vi "Video feed info class VI - states.vi"(0 "Video feed info in":refnum<class "Video feed info.lvclass">, 1 "States":T1, 2 "start path":path, 4 "Start/Stop":bool, 5 "error in (no error)":errorcluster, 6 "Slide Refnum":refnum<vi>) -> (8 "Image":T3(plugin-control), 9 "Start/Stop output":bool, 10 "file path":path, 11 "State output":T2(ring), 12 "Image Type":T4 items=["Grayscale (U8)", "Grayscale (I16)", "Grayscale (SGL)", "Complex (CSG)", "RGB (U32)", "HSL (U32)", "RGB (U64)", "Grayscale (U16)"], 13 "Current Frame":u32, 14 "Video feed info out":refnum<class "Video feed info.lvclass">, 15 "FPS":u32, 16 "width":u32, 17 "height":u32, 18 "Number of Frames":u32, 19 "error out":errorcluster)   [LabVIEW 2010, in "Video feed info.lvclass"]
uses:
  Video feed info.lvclass
  Controls/video control.ctl
  <vilib>/Vision/Image Controls.llb/IMAQ Image.ctl
  Video feed info.lvclass/Video feed info.ctl
  <vilib>/vision/Avi1.llb/AviRefnum.ctl
  <vilib>/vision/NI_Vision_Development_Module.lvlib
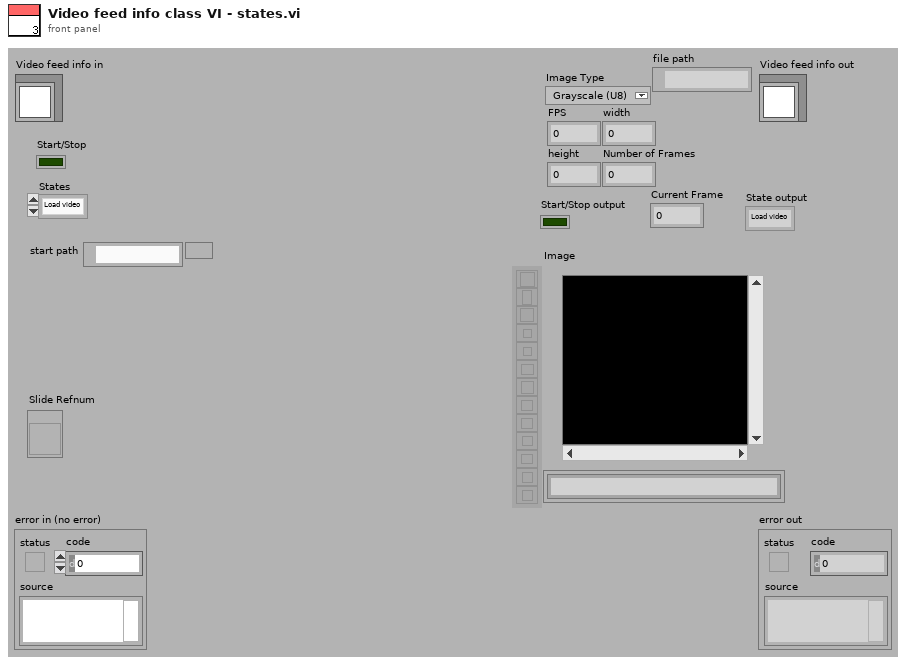
[diagram p1: front panel]
types:
  T1 = typedef "video control.ctl" = enum16{"Load video", "Idle", "Play", "Rewind", "Forward", "Dispose"}
  T2 = enum16{"Load video", "Idle", "Play", "Rewind", "Forward", "Dispose"}
  T3 = typedef "IMAQ Image.ctl" = refnum<image>
  T4 = typedef "Image Type" = u32
  T5 = cluster{"Number of Frames":u32, "Number of Frames":u32, "Number of Frames":u32}
  T6 = typedef "AviRefnum.ctl" = refnum<k1>
  T7 = cluster{"width":u32, "height":u32, "framesPerSecond":u32, "compressionFilter":string, "hasData":bool}
  T8 = cluster{"Higher Cursor value":u32, "Lower Cursor value":u32, "Current Frame":u32}
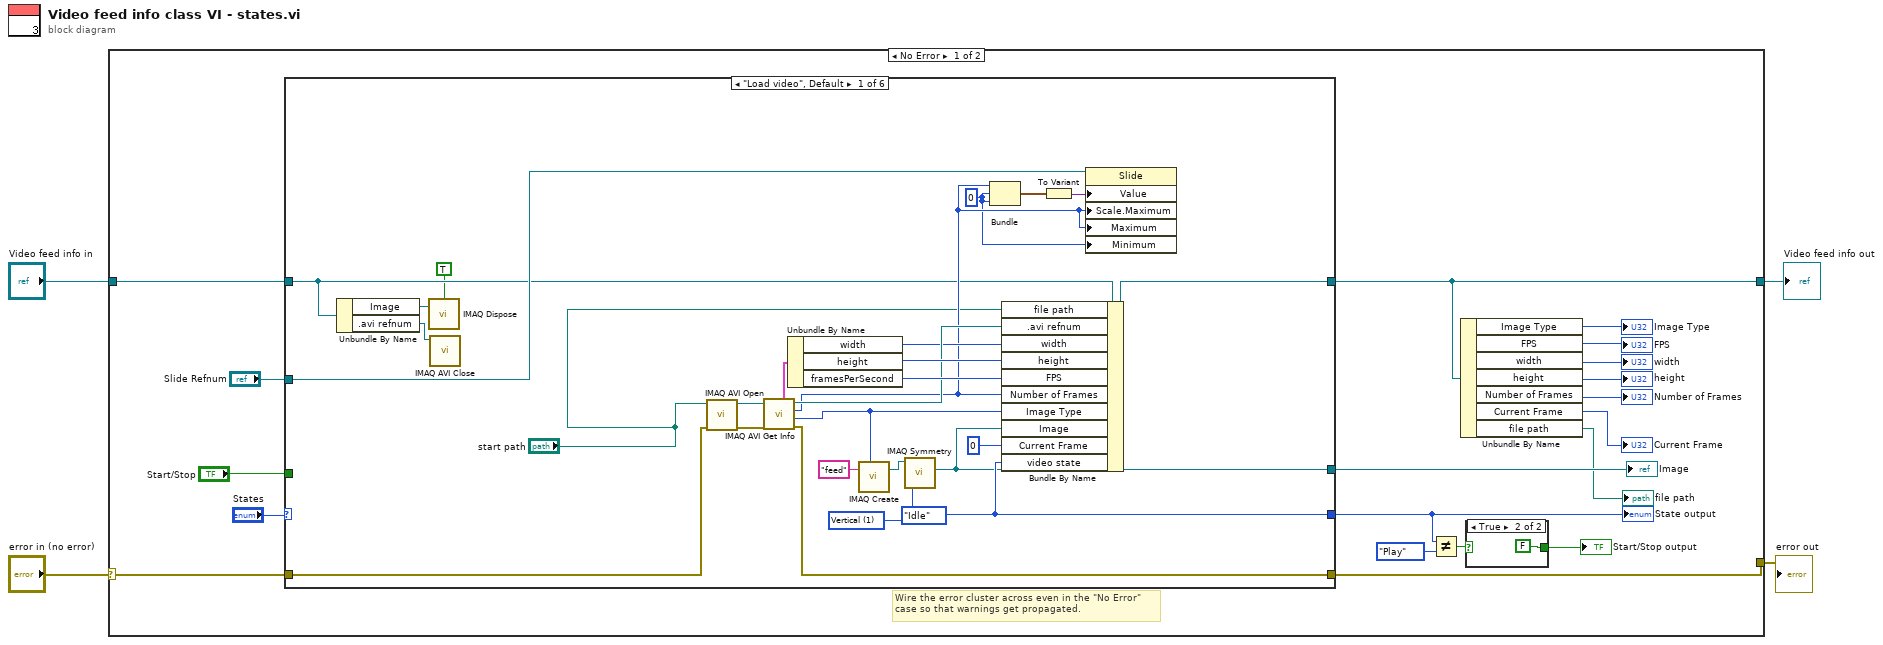
[diagram p0: block diagram]
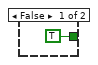
[diagram p2: hidden frame]
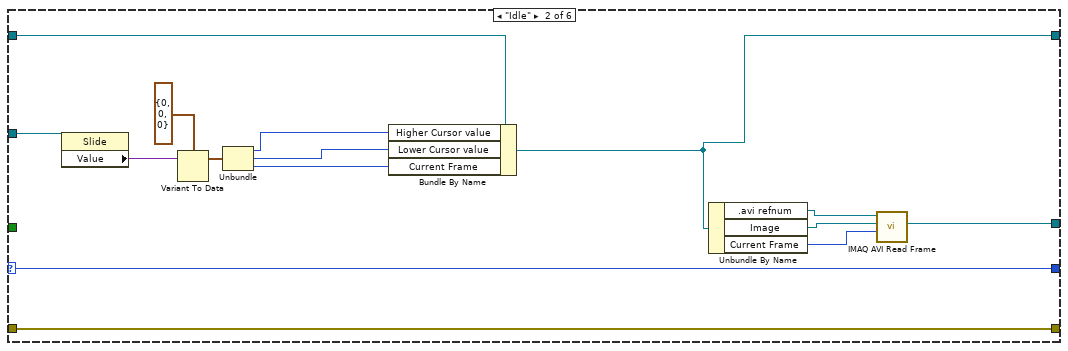
[diagram p3: hidden frame]
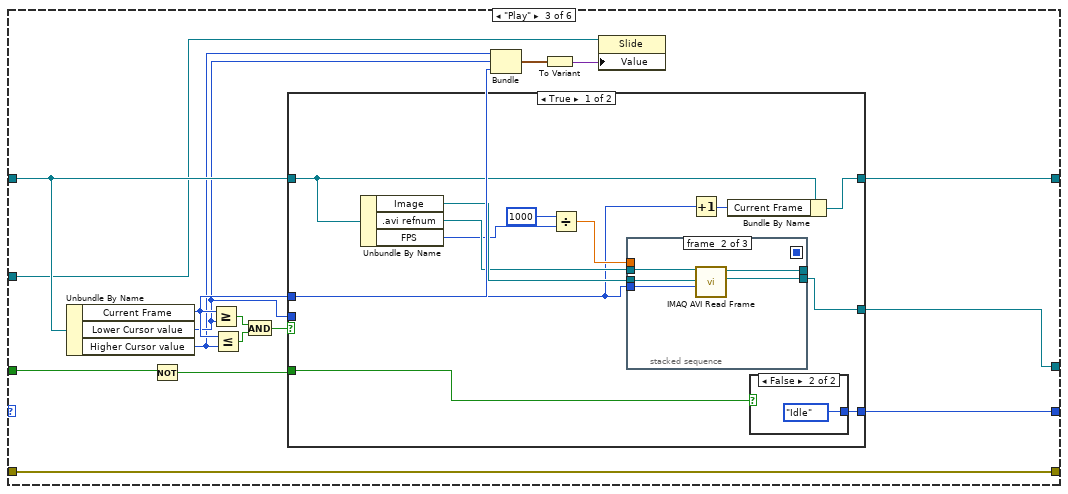
[diagram p4: hidden frame]
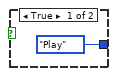
[diagram p5: hidden frame]
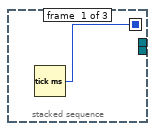
[diagram p6: hidden frame]
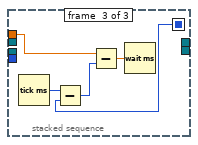
[diagram p7: hidden frame]
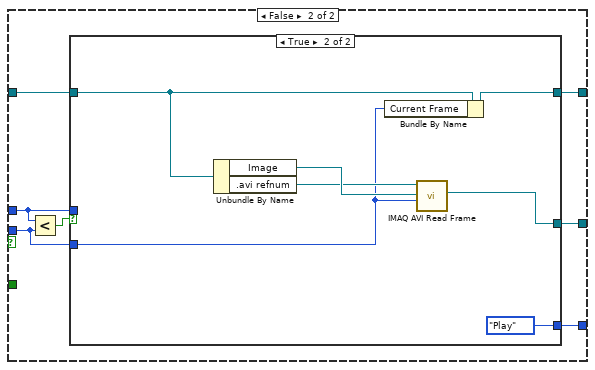
[diagram p8: hidden frame]
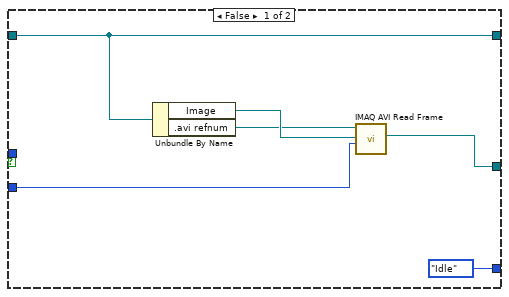
[diagram p9: hidden frame]
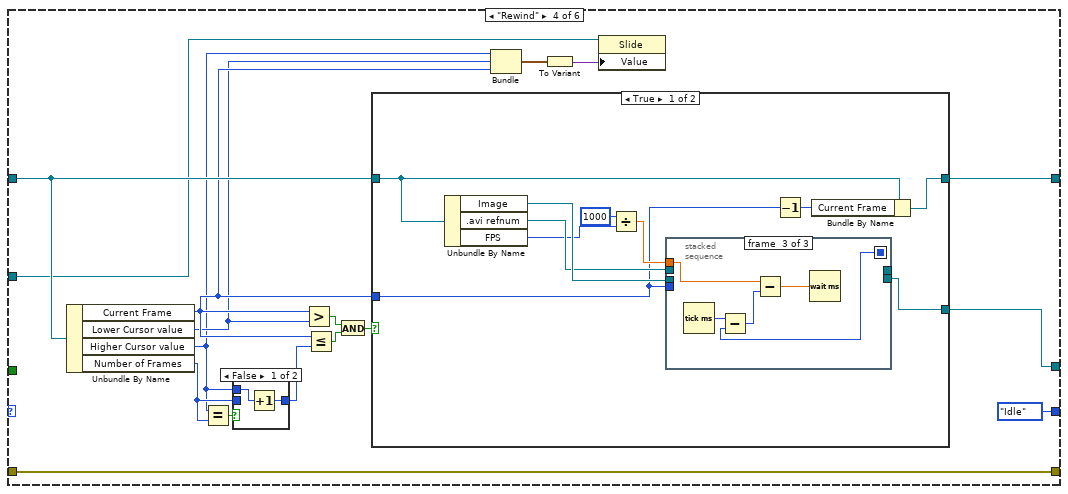
[diagram p10: hidden frame]
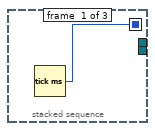
[diagram p12: hidden frame]
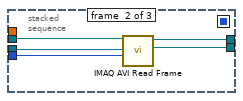
[diagram p13: hidden frame]
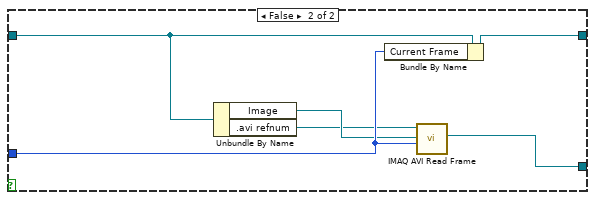
[diagram p14: hidden frame]
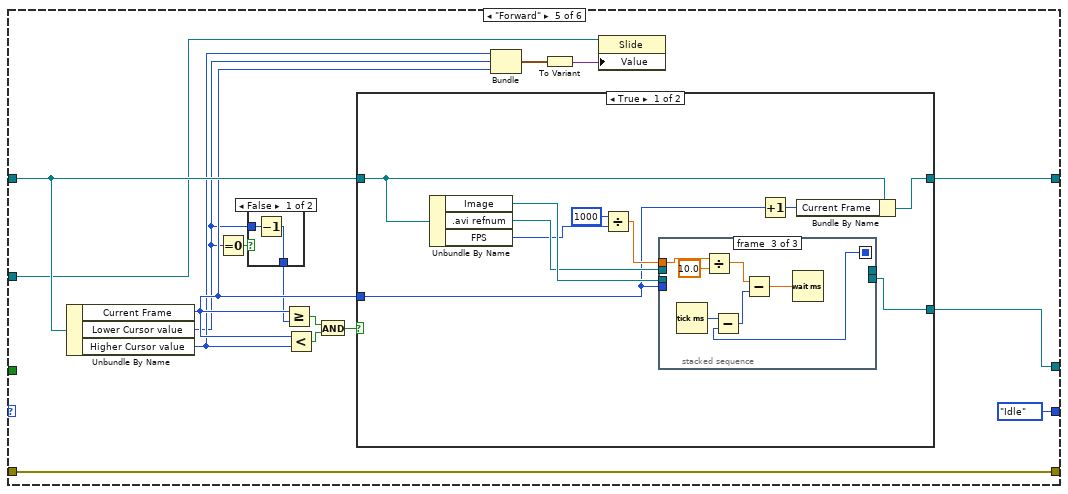
[diagram p15: hidden frame]
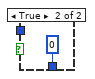
[diagram p16: hidden frame]
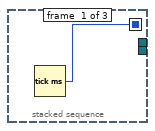
[diagram p17: hidden frame]
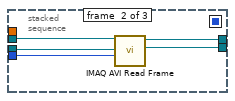
[diagram p18: hidden frame]
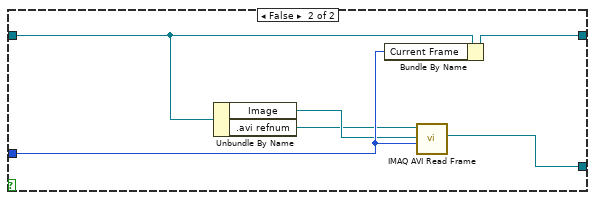
[diagram p19: hidden frame]
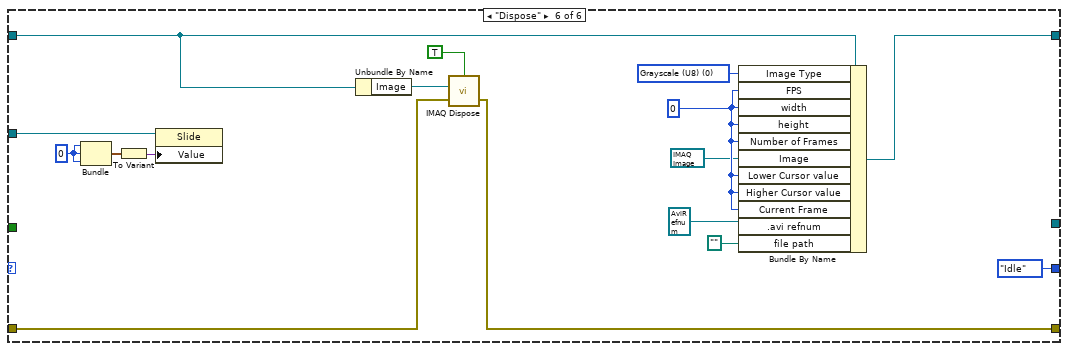
[diagram p20: hidden frame]
diagram:
  n1 = case shown="No Error" "error in (no error)" {
    selector: "error in (no error)" -> [w22 w241]
    tunnel: [w21 w241] -> w3
    tunnel: [w18 w240] -> w1
    tunnel: "Video feed info in" -> [w23 w240]
    frame No Error {
      # "Wire the error cluster across even in the \"No Error\"\ncase so that warnings get propagated."
      n2 = case shown="\"Load video\", Default" "States" {
        selector: "States" -> [_ w65 _ _ _ _]
        tunnel: w23 -> [w34 w66 w77 w140 w186 w234]
        tunnel: [w52 w63 w80 w142 w188 w233] -> w18
        tunnel: w22 -> [w49 w67 w78 w141 w187 w238]
        tunnel: [w46 w67 w78 w141 w187 w237] -> w21
        tunnel: [w28 w64 w68 w139 w185 _] -> w20
        tunnel: [w35 w65 w79 T2."Idle" ("Enum") T2."Idle" ("Enum") T2."Idle" ("Enum")] -> w9
        tunnel: "Start/Stop" -> [_ _ w76 _ _ _]
        tunnel: "Slide Refnum" -> [w38 w59 w72 w136 w182 w227]
        frame "Load video", Default {
          w26 = u32 1 items=["Horizontal", "Vertical", "Central", "1st Diagonal", "2nd Diagonal"] ("Type of Symmetry")
          w35 = T2."Idle" ("Enum")
          w31 = u32 0 ("Number of Frames")
          n3 = Unbundle By Name(w34) -> ("Image"=w33:T3, ".avi refnum"=w30:T6)
          n4 = call "IMAQ Dispose"("All Images? (No)"=TRUE, "Image"=w33) -> ()  [unwired: 4 in, 1 out]
          n5 = call "IMAQ AVI Close"("Avi Refnum"=w30) -> ()  [unwired: 10 in, 1 out]
          n6 = call "IMAQ AVI Open"("error in (no error)"=w49, "AVI Path"="start path") -> ("error out"=w48:errorcluster, "Avi Refnum"=w51:T6)  [unwired: 8 in]
          n7 = call "IMAQ AVI Get Info"("error in (no error)"=w48, "Avi Refnum"=w51) -> ("error out"=w46:errorcluster, "Image Type"=w45:T4, "Number of Frames"=w36:u32, "Avi Refnum (duplicate)"=w42:T6, "Frame Data"=w50:T7)  [unwired: 5 in]
          n8 = Unbundle By Name(w50) -> ("width"=w41:u32, "height"=w43:u32, "framesPerSecond"=w44:u32)
          n9 = call "IMAQ Create"("Image Name"="feed", "Image Type"=w45) -> ("New Image"=w27:T3)  [unwired: 3 in, 1 out]
          n10 = call "IMAQ Symmetry"("Type of Symmetry"=w26, "Image Src"=w27) -> ("Image Dst Out"=w28:T3)  [unwired: 3 in, 1 out]
          n11 = Bundle("Number of Frames"=w36, "Number of Frames"=w31, "Number of Frames"=w31) -> (w39:T5)  [unwired: 1 in]
          n12 = Bundle By Name(cluster=w34, "file path"="start path", ".avi refnum"=w42, "width"=w41, "height"=w43, "FPS"=w44, "Number of Frames"=w36, "Image Type"=w45, "Image"=w28, "Current Frame"=u32 0, "video state"=w35) -> (w52:refnum<class "Video feed info.lvclass">)
          n13 = To Variant(anything=w39) -> (Variant=w37:variant)
          n14 = property class="Slide"(reference=w38, "Value"=w37, "Scale.Maximum"=w36, "Maximum"=w36, "Minimum"=w31) -> ()  [unwired: 1 in, 2 out]
        }
        frame "Idle" {
          n15 = property class="Slide"(reference=w59) -> ("Value"=w58:variant)  [unwired: 1 in, 2 out]
          n16 = Variant To Data(Variant=w58, type=T5 {"Number of Frames"=0, "Number of Frames"=0, "Number of Frames"=0} ("cluster")) -> (data=w56:T5)  [unwired: 1 in, 1 out]
          n17 = Unbundle(w56) -> ("Number of Frames"=w54:u32, "Number of Frames"=w53:u32, "Number of Frames"=w55:u32)
          n18 = Bundle By Name(cluster=w66, "Higher Cursor value"=w54, "Lower Cursor value"=w53, "Current Frame"=w55) -> (w63:refnum<class "Video feed info.lvclass">)
          n19 = Unbundle By Name(w63) -> (".avi refnum"=w62:T6, "Image"=w61:T3, "Current Frame"=w60:u32)
          n20 = call "IMAQ AVI Read Frame"("Frame Number"=w60, "Image"=w61, "Avi Refnum"=w62) -> ("Image Out"=w64:T3)  [unwired: 5 in, 3 out]
        }
        frame "Play" {
          n21 = Unbundle By Name(w77) -> ("Current Frame"=w71:u32, "Lower Cursor value"=w70:u32, "Higher Cursor value"=w69:u32)
          n22 = Not(x=w76) -> (.not. x?=w75:bool)
          n23 = Greater Or Equal?(x=w71, y=w70) -> (x >= y?=w82:bool)
          n24 = Less Or Equal?(x=w71, y=w69) -> (x <= y?=w83:bool)
          n25 = And(x=w82, y=w83) -> (x .and. y?=w81:bool)
          n26 = case shown="True" w81 {
            tunnel: w77 -> [w93 w113]
            tunnel: w71 -> [w85 w109]
            tunnel: [w92 w111] -> w80
            tunnel: [w91 w115] -> w68
            tunnel: [w87 w114] -> w79
            tunnel: w75 -> [w86 _]
            tunnel: w70 -> [_ w110]
            frame True {
              n27 = Unbundle By Name(w93) -> ("Image"=w95:T3, ".avi refnum"=w94:T6, "FPS"=w89:u32)
              n28 = Divide(x=u32 1000, y=w89) -> (x/y=w88:dbl)
              n29 = stacked-sequence {
                seq-local: [w98 _ _] -> [_ _ w106]
                tunnel: w94 -> [_ w103 _]
                tunnel: w95 -> [_ w102 _]
                tunnel: [_ w101 _] -> _
                tunnel: [_ w100 _] -> w91
                tunnel: w88 -> [_ _ w108]
                tunnel: w85 -> [_ w99 _]
                frame #0 {
                  n30 = Tick Count (ms)() -> (millisecond timer value=w98:u32)
                }
                frame #1 {
                  n31 = call "IMAQ AVI Read Frame"("Frame Number"=w99, "Image"=w102, "Avi Refnum"=w103) -> ("Image Out"=w100:T3, "Avi Refnum (duplicate)"=w101:T6)  [unwired: 5 in, 2 out]
                }
                frame #2 {
                  n32 = Tick Count (ms)() -> (millisecond timer value=w107:u32)
                  n33 = Subtract(x=w107, y=w106) -> (x-y=w105:u32)
                  n34 = Subtract(x=w108, y=w105) -> (x-y=w104:dbl)
                  n35 = Wait (ms)(milliseconds to wait=w104) -> ()  [unwired: 1 out]
                }
              }
              n36 = Increment(x=w85) -> (x+1=w84:u32)
              n37 = Bundle By Name(cluster=w93, "Current Frame"=w84) -> (w92:refnum<class "Video feed info.lvclass">)
              n38 = case shown="False" w86 {
                tunnel: [T2."Play" ("Enum") T2."Idle" ("Enum")] -> w87
                frame True {
                }
                frame False {
                }
              }
            }
            frame False {
              n39 = Less?(x=w109, y=w110) -> (x < y?=w112:bool)
              n40 = case shown="True" w112 {
                tunnel: [w119 w126] -> w115
                tunnel: [T2."Idle" ("Enum") T2."Play" ("Enum")] -> w114
                tunnel: w113 -> [w118 w125]
                tunnel: [w118 w124] -> w111
                tunnel: w110 -> [w117 w123]
                tunnel: w109 -> [_ _]
                frame False {
                  n41 = Unbundle By Name(w118) -> ("Image"=w121:T3, ".avi refnum"=w120:T6)
                  n42 = call "IMAQ AVI Read Frame"("Frame Number"=w117, "Image"=w121, "Avi Refnum"=w120) -> ("Image Out"=w119:T3)  [unwired: 5 in, 3 out]
                }
                frame True {
                  n43 = Unbundle By Name(w125) -> ("Image"=w128:T3, ".avi refnum"=w127:T6)
                  n44 = Bundle By Name(cluster=w125, "Current Frame"=w123) -> (w124:refnum<class "Video feed info.lvclass">)
                  n45 = call "IMAQ AVI Read Frame"("Frame Number"=w123, "Image"=w128, "Avi Refnum"=w127) -> ("Image Out"=w126:T3)  [unwired: 5 in, 3 out]
                }
              }
            }
          }
          n46 = Bundle("Higher Cursor value"=w69, "Lower Cursor value"=w70, "Current Frame"=w71) -> (w74:T8)  [unwired: 1 in]
          n47 = To Variant(anything=w74) -> (Variant=w73:variant)
          n48 = property class="Slide"(reference=w72, "Value"=w73) -> ()  [unwired: 1 in, 2 out]
        }
        frame "Rewind" {
          n49 = Unbundle By Name(w140) -> ("Current Frame"=w135:u32, "Lower Cursor value"=w133:u32, "Higher Cursor value"=w129:u32, "Number of Frames"=w131:u32)
          n50 = Equal?(x=w129, y=w131) -> (x = y?=w132:bool)
          n51 = case shown="False" w132 {
            tunnel: w131 -> [_ w148]
            tunnel: [w147 w148] -> w130
            tunnel: w129 -> [w146 _]
            frame False {
              n52 = Increment(x=w146) -> (x+1=w147:u32)
            }
            frame True {
            }
          }
          n53 = Greater?(x=w135, y=w133) -> (0:w144:bool)
          n54 = Less Or Equal?(x=w135, y=w130) -> (x <= y?=w145:bool)
          n55 = And(x=w144, y=w145) -> (x .and. y?=w143:bool)
          n56 = case shown="True" w143 {
            tunnel: w140 -> [w156 w174]
            tunnel: w135 -> [w150 w172]
            tunnel: [w155 w173] -> w142
            tunnel: [w154 w175] -> w139
            frame True {
              n57 = Unbundle By Name(w156) -> ("Image"=w158:T3, ".avi refnum"=w157:T6, "FPS"=w152:u32)
              n58 = Divide(x=u32 1000, y=w152) -> (x/y=w151:dbl)
              n59 = stacked-sequence {
                seq-local: [w159 _ _] -> [_ _ w168]
                tunnel: w157 -> [_ w164 _]
                tunnel: w158 -> [_ w163 _]
                tunnel: [_ w162 _] -> _
                tunnel: [_ w161 _] -> w154
                tunnel: w151 -> [_ _ w166]
                tunnel: w150 -> [_ w160 _]
                frame #0 {
                  n60 = Tick Count (ms)() -> (millisecond timer value=w159:u32)
                }
                frame #1 {
                  n61 = call "IMAQ AVI Read Frame"("Frame Number"=w160, "Image"=w163, "Avi Refnum"=w164) -> ("Image Out"=w161:T3, "Avi Refnum (duplicate)"=w162:T6)  [unwired: 5 in, 2 out]
                }
                frame #2 {
                  n62 = Tick Count (ms)() -> (millisecond timer value=w169:u32)
                  n63 = Subtract(x=w169, y=w168) -> (x-y=w167:u32)
                  n64 = Subtract(x=w166, y=w167) -> (x-y=w165:dbl)
                  n65 = Wait (ms)(milliseconds to wait=w165) -> ()  [unwired: 1 out]
                }
              }
              n66 = Decrement(x=w150) -> (x-1=w149:u32)
              n67 = Bundle By Name(cluster=w156, "Current Frame"=w149) -> (w155:refnum<class "Video feed info.lvclass">)
            }
            frame False {
              n68 = Unbundle By Name(w174) -> ("Image"=w171:T3, ".avi refnum"=w170:T6)
              n69 = Bundle By Name(cluster=w174, "Current Frame"=w172) -> (w173:refnum<class "Video feed info.lvclass">)
              n70 = call "IMAQ AVI Read Frame"("Frame Number"=w172, "Image"=w171, "Avi Refnum"=w170) -> ("Image Out"=w175:T3)  [unwired: 5 in, 3 out]
            }
          }
          n71 = Bundle("Higher Cursor value"=w129, "Lower Cursor value"=w133, "Current Frame"=w135) -> (w138:T8)  [unwired: 1 in]
          n72 = To Variant(anything=w138) -> (Variant=w137:variant)
          n73 = property class="Slide"(reference=w136, "Value"=w137) -> ()  [unwired: 1 in, 2 out]
        }
        frame "Forward" {
          n74 = Unbundle By Name(w186) -> ("Current Frame"=w181:u32, "Lower Cursor value"=w177:u32, "Higher Cursor value"=w179:u32)
          n75 = Equal To 0?(x=w177) -> (x = 0?=w178:bool)
          n76 = case shown="False" w178 {
            tunnel: w177 -> [w193 _]
            tunnel: [w192 u32 0] -> w176
            frame False {
              n77 = Decrement(x=w193) -> (x-1=w192:u32)
            }
            frame True {
            }
          }
          n78 = Greater Or Equal?(x=w181, y=w176) -> (x >= y?=w190:bool)
          n79 = Less?(x=w181, y=w179) -> (x < y?=w191:bool)
          n80 = And(x=w190, y=w191) -> (x .and. y?=w189:bool)
          n81 = case shown="True" w189 {
            tunnel: w186 -> [w202 w222]
            tunnel: w181 -> [w196 w220]
            tunnel: [w201 w221] -> w188
            tunnel: [w200 w223] -> w185
            frame True {
              n82 = Unbundle By Name(w202) -> ("Image"=w204:T3, ".avi refnum"=w203:T6, "FPS"=w198:u32)
              n83 = Divide(x=u32 1000, y=w198) -> (x/y=w197:dbl)
              n84 = stacked-sequence {
                seq-local: [w205 _ _] -> [_ _ w216]
                tunnel: w203 -> [_ w210 _]
                tunnel: w204 -> [_ w209 _]
                tunnel: [_ w208 _] -> _
                tunnel: [_ w207 _] -> w200
                tunnel: w197 -> [_ _ w214]
                tunnel: w196 -> [_ w206 _]
                frame #0 {
                  n85 = Tick Count (ms)() -> (millisecond timer value=w205:u32)
                }
                frame #1 {
                  n86 = call "IMAQ AVI Read Frame"("Frame Number"=w206, "Image"=w209, "Avi Refnum"=w210) -> ("Image Out"=w207:T3, "Avi Refnum (duplicate)"=w208:T6)  [unwired: 5 in, 2 out]
                }
                frame #2 {
                  n87 = Tick Count (ms)() -> (millisecond timer value=w217:u32)
                  n88 = Divide(x=w214, y=10.0) -> (x/y=w212:dbl)
                  n89 = Subtract(x=w217, y=w216) -> (x-y=w215:u32)
                  n90 = Subtract(x=w212, y=w215) -> (x-y=w213:dbl)
                  n91 = Wait (ms)(milliseconds to wait=w213) -> ()  [unwired: 1 out]
                }
              }
              n92 = Increment(x=w196) -> (x+1=w195:u32)
              n93 = Bundle By Name(cluster=w202, "Current Frame"=w195) -> (w201:refnum<class "Video feed info.lvclass">)
            }
            frame False {
              n94 = Unbundle By Name(w222) -> ("Image"=w219:T3, ".avi refnum"=w218:T6)
              n95 = Bundle By Name(cluster=w222, "Current Frame"=w220) -> (w221:refnum<class "Video feed info.lvclass">)
              n96 = call "IMAQ AVI Read Frame"("Frame Number"=w220, "Image"=w219, "Avi Refnum"=w218) -> ("Image Out"=w223:T3)  [unwired: 5 in, 3 out]
            }
          }
          n97 = Bundle("Higher Cursor value"=w179, "Lower Cursor value"=w177, "Current Frame"=w181) -> (w184:T8)  [unwired: 1 in]
          n98 = To Variant(anything=w184) -> (Variant=w183:variant)
          n99 = property class="Slide"(reference=w182, "Value"=w183) -> ()  [unwired: 1 in, 2 out]
        }
        frame "Dispose" {
          w224 = u32 0 ("FPS")
          w230 = u32 0 ("FPS")
          w231 = T4 0 items=["Grayscale (U8)", "Grayscale (I16)", "Grayscale (SGL)", "Complex (CSG)", "RGB (U32)", "HSL (U32)", "RGB (U64)", "Grayscale (U16)"] ("Image Type")
          n100 = Bundle("FPS"=w224, "FPS"=w224, "FPS"=w224) -> (w226:cluster{"FPS":u32, "FPS":u32, "FPS":u32})  [unwired: 1 in]
          n101 = To Variant(anything=w226) -> (Variant=w225:variant)
          n102 = property class="Slide"(reference=w227, "Value"=w225) -> ()  [unwired: 1 in, 2 out]
          n103 = Unbundle By Name(w234) -> ("Image"=w239:T3)
          n104 = call "IMAQ Dispose"("All Images? (No)"=TRUE, "Image"=w239, "error in (no error)"=w238) -> ("error out"=w237:errorcluster)  [unwired: 3 in]
          n105 = Bundle By Name(cluster=w234, "Image Type"=w231, "FPS"=w230, "width"=w230, "height"=w230, "Number of Frames"=w230, "Image"=T3 refnum, "Lower Cursor value"=w230, "Higher Cursor value"=w230, "Current Frame"=w230, ".avi refnum"=T6 refnum, "file path"=path "") -> (w233:refnum<class "Video feed info.lvclass">)
        }
      }
      "Image" <- w20
      "State output" <- w9
      n106 = Not Equal?(x=w9, y=T2."Play" ("Enum")) -> (x != y?=w10:bool)
      n107 = Unbundle By Name(w18) -> ("Image Type"=→"Image Type":T4, "FPS"=→"FPS":u32, "width"=→"width":u32, "height"=→"height":u32, "Number of Frames"=→"Number of Frames":u32, "Current Frame"=→"Current Frame":u32, "file path"=→"file path":path)
      n108 = case shown="True" w10 {
        tunnel: [TRUE FALSE] -> w8
        frame False {
        }
        frame True {
        }
      }
      "Start/Stop output" <- w8
    }
    frame Error {
    }
  }
  "error out" <- w3
  "Video feed info out" <- w1
